vi "VITester API.vi"() -> ()   [LabVIEW 2020]
uses:
  <vilib>/addons/_JKI Toolkits/VI Tester/VI Tester API.llb/Run Tests (Path).vi
  <vilib>/addons/_JKI Toolkits/VI Tester/VI Tester API.llb/VI Tester API.lvlib
panel:
  out "test details":string
  out "Test Time [ms]":u32
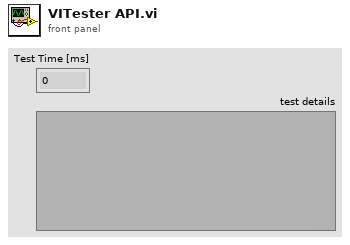
[diagram p1: front panel]
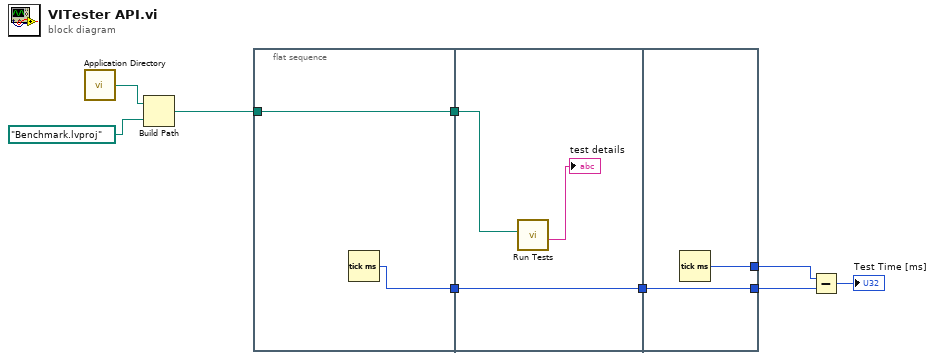
[diagram p0: block diagram]
diagram:
  n1 = call <vilib>:"Application Directory.vi"() -> ("Application Directory"=w9:path)
  n2 = Build Path(base path=w9, name or relative path=path "Benchmark.lvproj" ("Path")) -> (appended path=w1:path)
  n3 = flat-sequence {
    tunnel: [w11] -> w7
    tunnel: w1 -> [w11]
    tunnel: [w10] -> w5
    tunnel: w7 -> [w13]
    tunnel: w5 -> [w14]
    tunnel: [w14] -> w4
    tunnel: [w16] -> w6
    tunnel: w4 -> [w15]
    tunnel: [w15] -> w3
    frame #0 {
      n4 = Tick Count (ms)() -> (millisecond timer value=w10:u32)
    }
    frame #1 {
      n5 = call-poly <vilib>:"Run Tests.vi"("Test Path"=w13) -> ("test details"=→"test details":string)  [unwired: 8 in, 2 out]
    }
    frame #2 {
      n6 = Tick Count (ms)() -> (millisecond timer value=w16:u32)
    }
  }
  n7 = Subtract(x=w6, y=w3) -> (x-y=→"Test Time [ms]":u32)
